vi "Diff_Drive_System_Get_Speed.vi"() -> (1 "Right Speed FT/S":dbl, 3 "Left Speed FT/S":dbl)   [LabVIEW 2019]
uses:
  Diff_Drive_System_Globals.vi
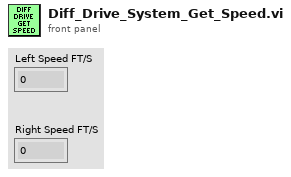
[diagram p1: front panel]
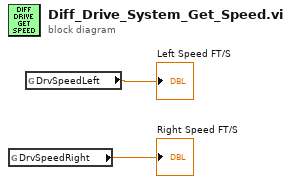
[diagram p0: block diagram]
diagram:
  n1 = global read "Diff_Drive_System_Globals.vi" "DrvSpeedRight"() -> (→"Right Speed FT/S":dbl)
  n2 = global read "Diff_Drive_System_Globals.vi" "DrvSpeedLeft"() -> (→"Left Speed FT/S":dbl)
